vi "Init Nontarget Histogram.vi"(8 "error in (no error)":errorcluster, 11 "Tosca in":refnum<class "Parameters.lvclass">) -> (0 "error out":errorcluster, 2 "Data":T1, 3 "Tosca out":refnum<class "Parameters.lvclass">)   [LabVIEW 2015, in "Parameters.lvclass"]
uses:
  Parameters.lvclass
  Histogram Data.ctl
  Parameters.lvclass/Parameters.ctl
  State/State.lvclass/State.ctl
  Termination/Termination.lvclass/Termination.ctl
  Timeout/Timeout.lvclass/Timeout.ctl
  Termination/Read Result.vi
  Termination/Read Color.vi
  Timeout/Read Result.vi
  Timeout/Read Color.vi
  State/Read Name.vi
  State/Read Term.vi
  State/Read Timeouts.vi
  Termination/Termination.lvclass
  Timeout/Timeout.lvclass
  State/State.lvclass
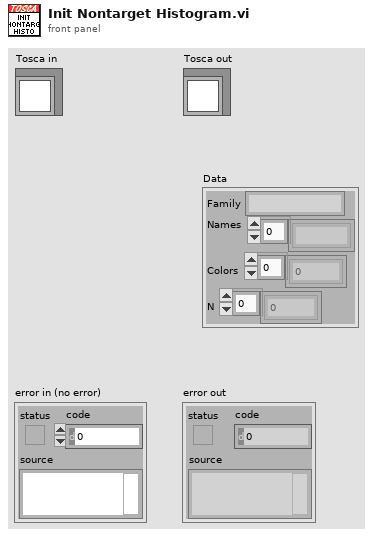
[diagram p1: front panel]
types:
  T1 = typedef "Parameters.lvclass/Histogram Data.ctl" = cluster{"Family":string, "Names":string[], "Colors":u32[], "N":i32[]}
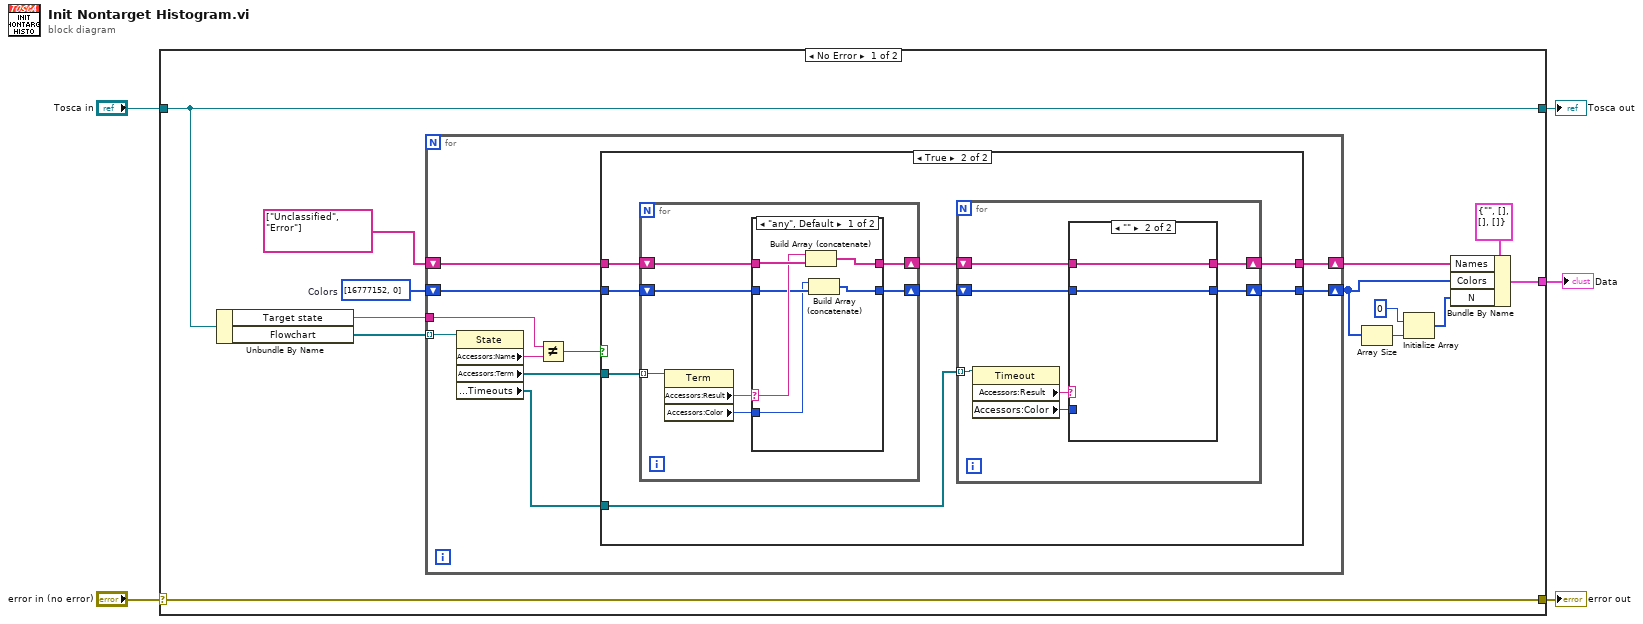
[diagram p0: block diagram]
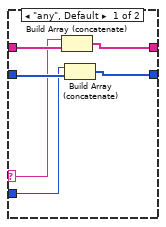
[diagram p3: hidden frame]
diagram:
  n1 = case shown="No Error" "error in (no error)" {
    selector: "error in (no error)" -> [w18 w70]
    tunnel: [w18 w70] -> w4
    tunnel: [w17 w69] -> w2
    tunnel: "Tosca in" -> [w17 w69]
    tunnel: [w6 _] -> w1
    frame No Error {
      w13 = u32[] [16777152, 0]  # Colors
      n2 = Unbundle By Name(w17) -> ("Target state"=w15:string, "Flowchart"=w16:refnum<class "State.lvclass">[])
      n3 = for {
        tunnel: w16 -> [w27] mode=indexing
        tunnel: w15 -> [w24]
        shift-right: [w22] -> w11
        shift-left: string[] ["Unclassified", "Error"] -> [w21]
        shift-right: [w19] -> w10
        shift-left: w13 -> [w20]
        n4 = property class="State"(reference=w27) -> ("Accessors:Name"=w25:string, "Accessors:Term"=w26:refnum<class "Termination.lvclass">[], "Accessors:Timeouts"=w28:refnum<class "Timeout.lvclass">[])  [unwired: 1 in, 2 out]
        n5 = Not Equal?(x=w24, y=w25) -> (x != y?=w23:bool)
        n6 = case shown="True" w23 {
          tunnel: w28 -> [_ w38]
          tunnel: w26 -> [_ w37]
          tunnel: [w30 w32] -> w22
          tunnel: w21 -> [w30 w36]
          tunnel: w20 -> [w29 w35]
          tunnel: [w29 w31] -> w19
          frame False {
          }
          frame True {
            n7 = for {
              tunnel: w37 -> [w60] mode=indexing
              shift-right: [w55] -> w34
              shift-left: w36 -> [w57]
              shift-right: [w54] -> w33
              shift-left: w35 -> [w56]
              n8 = property class="Term"(reference=w60) -> ("Accessors:Result"=w59:string, "Accessors:Color"=w58:u32)  [unwired: 1 in, 2 out]
              n9 = case shown="\"any\", Default" w59 {
                selector: w59 -> [w65 _]
                tunnel: w58 -> [w62 _]
                tunnel: w57 -> [w66 w68]
                tunnel: w56 -> [w63 w67]
                tunnel: [w64 w68] -> w55
                tunnel: [w61 w67] -> w54
                frame "any", Default {
                  n10 = Build Array (concatenate)(w65, w66) -> (w64:string[])
                  n11 = Build Array (concatenate)(w62, w63) -> (w61:u32[])
                }
                frame "" {
                }
              }
            }
            n12 = for {
              tunnel: w38 -> [w45] mode=indexing
              shift-right: [w40] -> w32
              shift-left: w34 -> [w42]
              shift-right: [w39] -> w31
              shift-left: w33 -> [w41]
              n13 = property class="Timeout"(reference=w45) -> ("Accessors:Result"=w44:string, "Accessors:Color"=w43:u32)  [unwired: 1 in, 2 out]
              n14 = case shown="\"\"" w44 {
                selector: w44 -> [w49 _]
                tunnel: w43 -> [w48 _]
                tunnel: w42 -> [w51 w53]
                tunnel: w41 -> [w50 w52]
                tunnel: [w47 w53] -> w40
                tunnel: [w46 w52] -> w39
                frame "any", Default {
                  n15 = Build Array (concatenate)(w49, w51) -> (w47:string[])
                  n16 = Build Array (concatenate)(w48, w50) -> (w46:u32[])
                }
                frame "" {
                }
              }
            }
          }
        }
      }
      n17 = Array Size(array=w10) -> (size(s)=w9:i32)
      n18 = Initialize Array(0, w9) -> (w7:i32[])
      n19 = Bundle By Name(cluster=T1 {"Family"="", "Names"=[], "Colors"=[], "N"=[]} ("array"), "Names"=w11, "Colors"=w10, "N"=w7) -> (w6:T1)
    }
    frame Error {
    }
  }
  "error out" <- w4
  "Tosca out" <- w2
  "Data" <- w1
